vi "canvas_drawing_example.vi"() -> ()   [LabVIEW 2021]
panel:
  out "Position:Top":i32
  out "Position:Left":i32
  in  "new picture":picture
  out "CursLoc":cluster{"X":dbl, "Y":dbl}
  in  "stop":bool
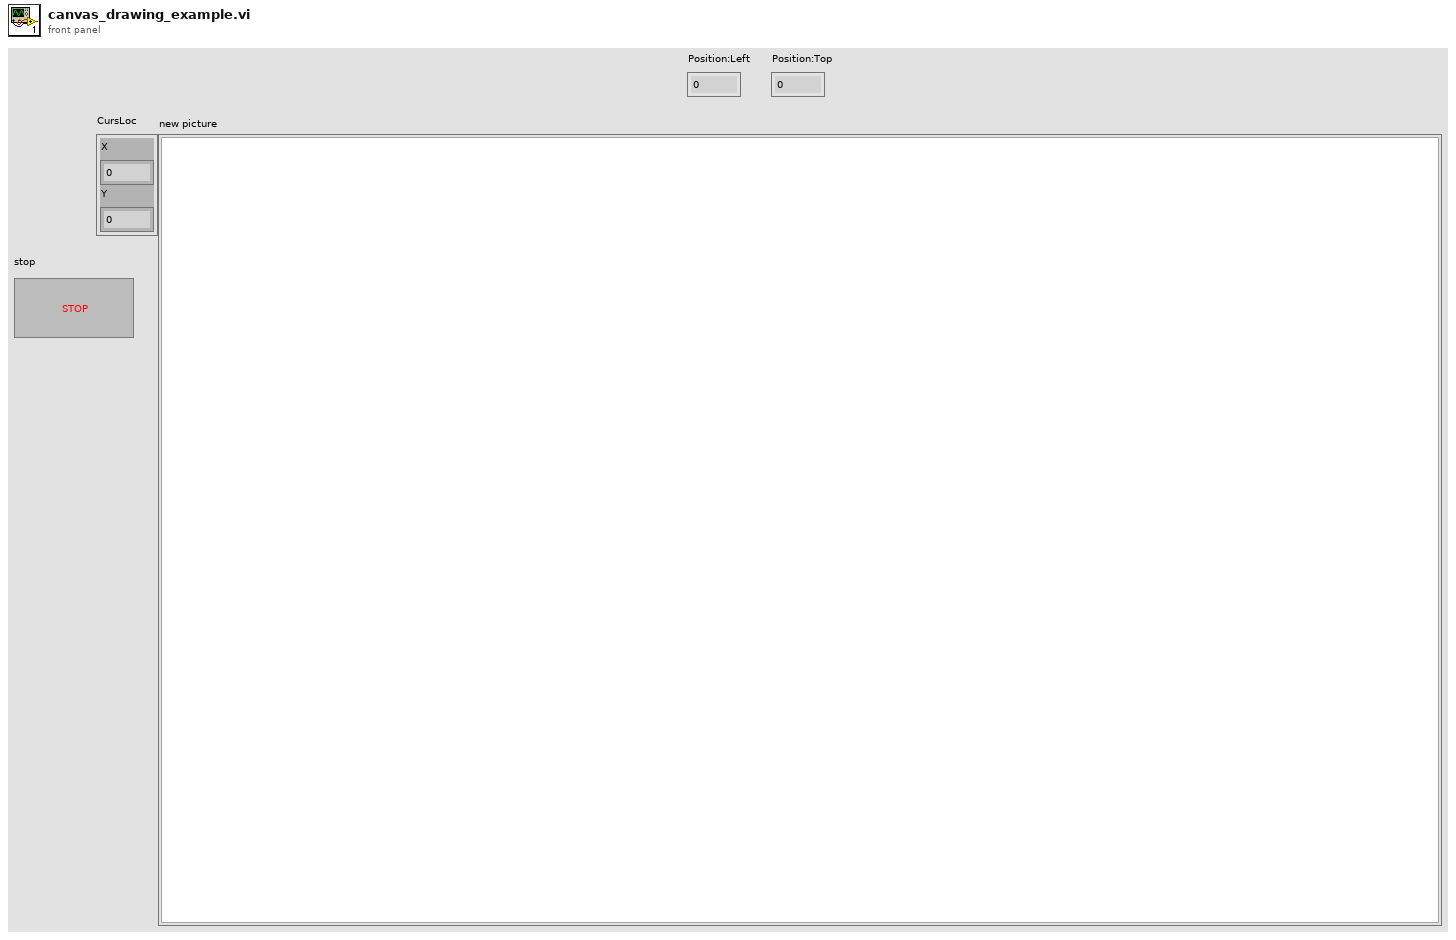
[diagram p1: front panel]
types:
  T1 = cluster{"Width":u16, "Style":enum32{"Solid", "Dash", "Dot", "DashDot", "DashDotDot"}}
  T2 = typedef "LVPoint32TypeDef.ctl" = cluster{"Horizontal":i32, "Vertical":i32}
  T3 = typedef "LVPositionTypeDef.ctl" = cluster{"Left":i32, "Top":i32}
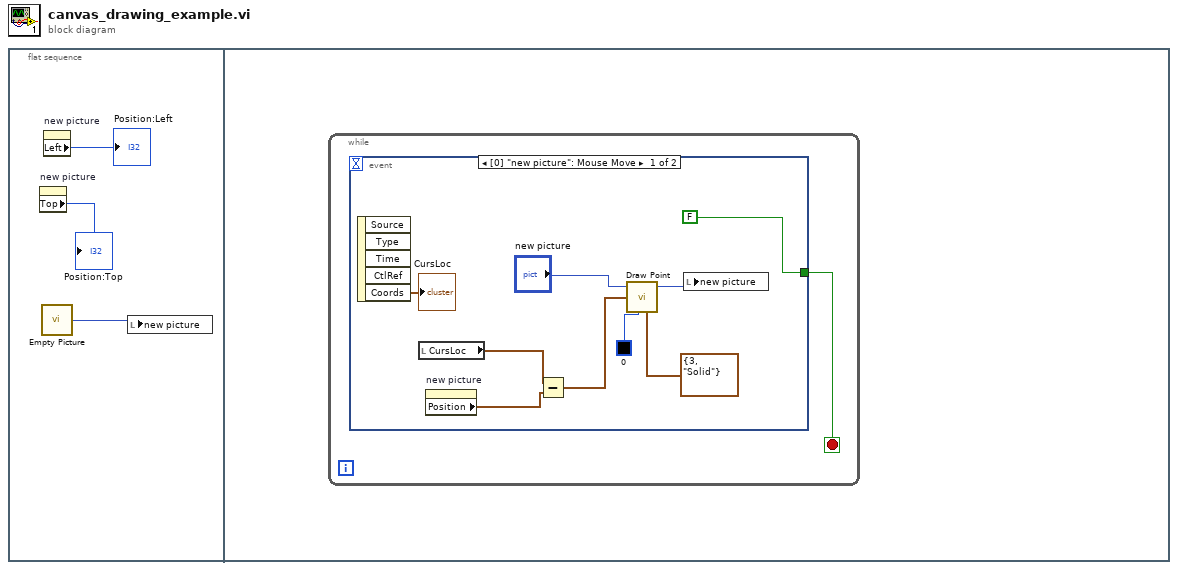
[diagram p0: block diagram]
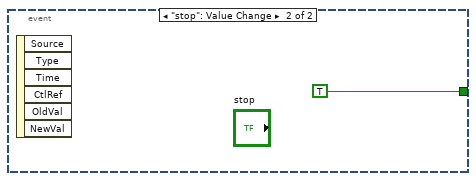
[diagram p2: hidden frame]
diagram:
  n1 = flat-sequence {
    frame #0 {
      n2 = property on="new picture" class="Pict"() -> ("Top"=→"Position:Top":i32)  [unwired: 2 in, 2 out]
      n3 = call "Empty Picture"() -> ("empty picture"=w3:picture)
      n4 = property on="new picture" class="Pict"() -> ("Left"=→"Position:Left":i32)  [unwired: 2 in, 2 out]
      n5 = local write "new picture"(w3) -> ()
    }
    frame #1 {
      n6 = while {
        stop <- w4 stop-if-true
        n7 = event shown="[0] \"new picture\": Mouse Move" {
          selector: _ -> [_ _]
          dyn-events: _ -> [_ _]
          timeout: _ -> [_ _]
          tunnel: [FALSE TRUE] -> w4
          event "new picture": Mouse Move {
            n8 = event-data() -> ("Coords"=→"CursLoc":T2)  [unwired: 1 in, 4 out]
            n9 = local read "CursLoc"() -> (w7:cluster{"X":dbl, "Y":dbl})
            n10 = property on="new picture" class="Pict"() -> ("Position"=w6:T3)  [unwired: 2 in, 2 out]
            n11 = Subtract(x=w7, y=w6) -> (x-y=w5:cluster{dbl, dbl})
            n12 = call <vilib>:"Draw Point.vi"("picture"="new picture", "point(x,y)"=w5, "color(black)"=u32 0, "pen"=T1 {"Width"=3, "Style"=enum."Solid"}) -> ("new picture"=w10:picture)  [unwired: 5 in]
            n13 = local write "new picture"(w10) -> ()
          }
          event "stop": Value Change {
            n14 = event-data() -> ()  [unwired: 1 in, 6 out]
          }
        }
      }
    }
  }
